vi "Slice Rows Cols.vi"(0 "Image_2d":i16[][](array[numeric]), 5 "error in (no error)":errorcluster, 7 "Slice Rows(T)/Cols(F)":bool=TRUE, 9 "Start Index":i32, 11 "Stop Index":i32) -> (14 "Image_2d_Slice":i16[][](array[numeric]), 19 "error out":errorcluster)   [LabVIEW 2016]
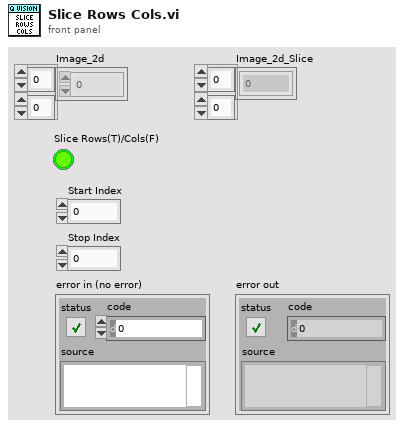
[diagram p1: front panel]
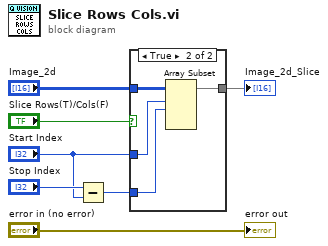
[diagram p0: block diagram]
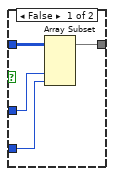
[diagram p2: hidden frame]
diagram:
  n1 = Subtract(x="Stop Index", y="Start Index") -> (x-y=w2:i32)
  n2 = case shown="True" "Slice Rows(T)/Cols(F)" {
    tunnel: "Image_2d" -> [w11 w15]
    tunnel: [w10 w14] -> w4
    tunnel: w2 -> [w8 w12]
    tunnel: "Start Index" -> [w9 w13]
    frame False {
      n3 = Array Subset(array=w11, index (col)=w9, length (col)=w8) -> (w10:i16[][])  [unwired: 2 in]
    }
    frame True {
      n4 = Array Subset(array=w15, index (row)=w13, length (row)=w12) -> (w14:i16[][])  [unwired: 2 in]
    }
  }
  "Image_2d_Slice" <- w4
  "error out" <- "error in (no error)"
